vi "Test Exec.vi"(5 "Chunk Size":i32, 7 "Sample Rate":i32, 8 "Shape":T2, 9 "Frequency":T3, 10 "Offset":T3, 11 "Amplitude":T3) -> (3 "Out":T1)   [LabVIEW 2022 SP3]
uses:
  <extravilib>/ChannelInstances/Flex-dbl/))Channel.ctl
  <extravilib>/ChannelInstances/Flex-t'FGen.lvlib-Shape.ctl'/))Channel.ctl
  Users/Localization Tester/Documents/LabVIEW Data/IlluminatedG/FlexBlocks/Workers/FGen/Shape.ctl
  <extravilib>/ChannelInstances/Flex-c(dbl,dbl,a[.](dbl))/))Channel.ctl
  Users/Localization Tester/Documents/LabVIEW Data/IlluminatedG/FlexBlocks/Workers/FGen/State.ctl
  FlexBlocks Support/Worker Action.ctl
  Users/Localization Tester/Documents/LabVIEW Data/IlluminatedG/FlexBlocks/Workers/FGen/Init.ctl
  Users/Localization Tester/Documents/LabVIEW Data/IlluminatedG/FlexBlocks/Workers/FGen/Tags.ctl
  f1ba7f41-6067-463b-82d1-95e17fac6f2e.vi
  Users/Localization Tester/Documents/LabVIEW Data/IlluminatedG/FlexBlocks/Workers/FGen/Work.vi
  <extravilib>/ChannelInstances/Messenger-t'FlexBlocks Support.lvlib-Execution Events.ctl'/Instantiate.vi
  FlexBlocks Support/FlexBlocks Support.lvlib
  Users/Localization Tester/Documents/LabVIEW Data/IlluminatedG/FlexBlocks/Workers/FGen/FGen.lvlib
  <extravilib>/ChannelInstances/Flex-dbl.lvlib
  <extravilib>/ChannelInstances/Flex-t'FGen.lvlib-Shape.ctl'.lvlib
  <extravilib>/ChannelInstances/Flex-c(dbl,dbl,a[.](dbl)).lvlib
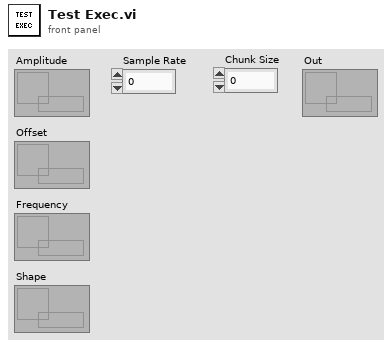
[diagram p1: front panel]
types:
  T1 = typedef "Flex-c(dbl,dbl,a[.](dbl)).lvlib/))Channel.ctl" = refnum<queue>
  T2 = typedef "Flex-t'FGen.lvlib-Shape.ctl'.lvlib/))Channel.ctl" = refnum<queue>
  T3 = typedef "Flex-dbl.lvlib/))Channel.ctl" = refnum<queue>
  T4 = typedef "FGen.lvlib/State.ctl" = cluster{"sampling info":cluster{"Fs":dbl, "#s":dbl}, "dx":dbl, "Delay":i32}
  T5 = typedef "Messenger-t'FlexBlocks Support.lvlib-Execution Events.ctl'.lvlib/))Channel.ctl" = refnum<queue>
  T6 = typedef "FlexBlocks Support.lvlib/Worker Block.ctl" = cluster{"Block Status":refnum<user-event>, "Command Queue":refnum<queue>, "Status":T7}
  T7 = typedef "FlexBlocks Support.lvlib/Block Status with Error.ctl" = cluster{"Block Status":T8, "Error":errorcluster}
  T8 = typedef "FlexBlocks Support.lvlib/Block Status.ctl" = cluster{"State":T9, "Next State":T9, "Runs":u32, "i":i32, "Init":bool, "Started":bool, "Closing":bool, "Step":bool, "Phase":T10, "Worker":string}
  T9 = typedef "FlexBlocks Support.lvlib/Block State.ctl" = enum16{"Idle", "Init", "Start", "Run", "Stop", "Close"}
  T10 = typedef "FlexBlocks Support.lvlib/Block Phase.ctl" = enum16{"N/A", "Read", "Work", "Write"}
  T11 = typedef "FlexBlocks Support.lvlib/Worker Action.ctl" = enum16{"Init", "Start", "Run", "Stop", "Close"}
  T12 = typedef "FGen.lvlib/Shape.ctl" = enum16{"Sine", "Square", "Triangle", "Saw"}
  T13 = typedef "FGen.lvlib/Init.ctl" = cluster{"Sample Rate":i32, "Chunk Size":i32}
  T14 = typedef "FGen.lvlib/Tags.ctl" = cluster{"Shape":T12, "Frequency":dbl, "Amplitude":dbl, "Offset":dbl}
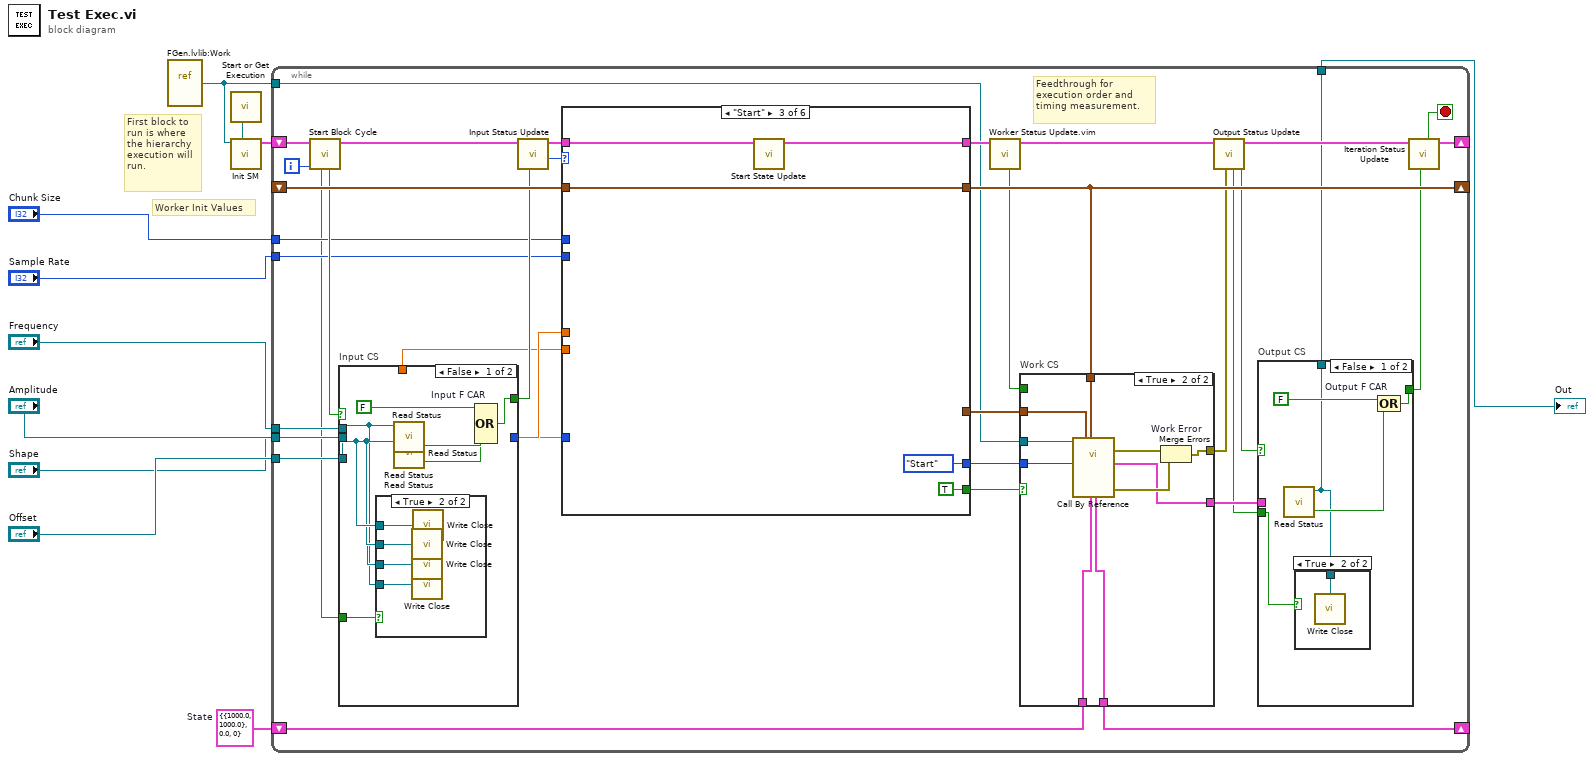
[diagram p0: block diagram]
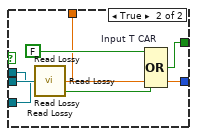
[diagram p3: hidden frame]
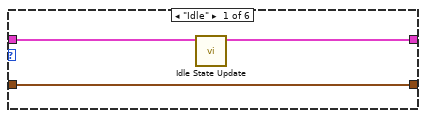
[diagram p4: hidden frame]
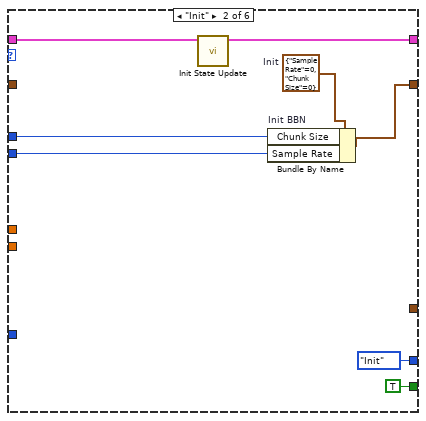
[diagram p5: hidden frame]
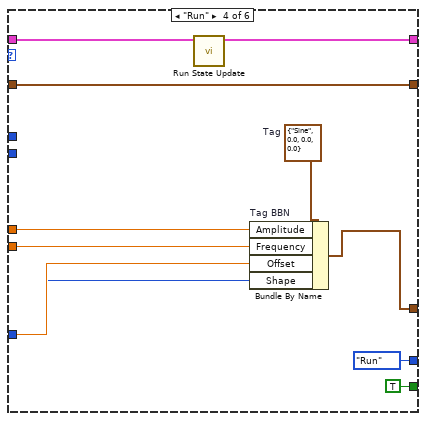
[diagram p6: hidden frame]
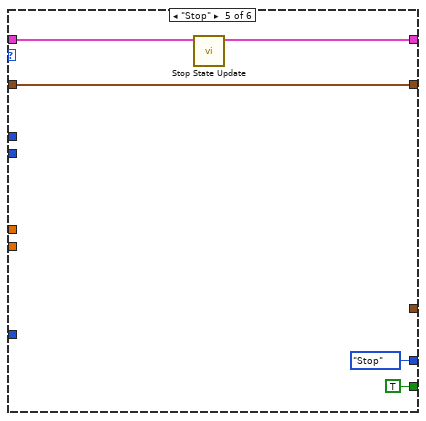
[diagram p7: hidden frame]
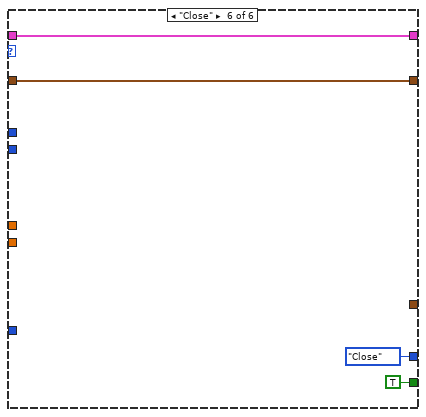
[diagram p8: hidden frame]
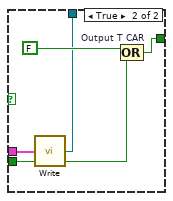
[diagram p10: hidden frame]
diagram:
  w11 = T4 {"sampling info"={"Fs"=1000.0, "#s"=1000.0}, "dx"=0.0, "Delay"=0}  # State
  # "First block to run is where the hierarchy execution will run."
  # "Worker Init Values"
  n1 = vi-ref "FGen.lvlib:Work.vi"() -> (w10:refnum<vi>)
  n2 = call "Start or Get Execution.vi"() -> ("Exec Events"=w9:T5)  [unwired: 11 in]
  n3 = call "Init SM.vi"("Exec Events"=w9, "Work VI"=w10) -> ("Worker Block"=w8:T6)  [unwired: 9 in]
  n4 = while {
    tunnel: w10 -> [w29]
    shift-right: [w48] -> _
    shift-left: w11 -> [w49]
    shift-right: [w34] -> _
    shift-left: w8 -> [w41]
    shift-right: [w45] -> _
    shift-left: _ -> [w46]
    tunnel: "Chunk Size" -> [w26]
    tunnel: "Sample Rate" -> [w25]
    tunnel: "Amplitude" -> [w24]
    tunnel: "Frequency" -> [w22]
    tunnel: "Offset" -> [w20]
    tunnel: "Shape" -> [w18]
    tunnel: [w16] -> w1
    i -> [w27]
    stop <- w32 stop-if-true
    # "Feedthrough for execution order and timing measurement."
    n5 = call "Start Block Cycle.vi"("i"=w27, "Worker Block In"=w41) -> ("Worker Block"=w40:T6, "Do Read"=w43:bool, "Close"=w14:bool)  [unwired: 7 in]
    n6 = case "Input CS" shown="False" w43 {
      tunnel: [w60 w78] -> w39
      tunnel: w24 -> [w50 w76]
      tunnel: [_ w74] -> w23
      tunnel: w22 -> [w51 w73]
      tunnel: [_ w71] -> w21
      tunnel: w20 -> [w52 w70]
      tunnel: [_ w68] -> w19
      tunnel: w18 -> [w53 w67]
      tunnel: [_ w65] -> w17
      tunnel: w14 -> [w54 _]
      frame False {
        n7 = case shown="True" w54 {
          tunnel: w53 -> [_ w64]
          tunnel: w52 -> [_ w63]
          tunnel: w51 -> [_ w62]
          tunnel: w50 -> [_ w61]
          frame False {
          }
          frame True {
            n8 = call <extravilib>:"Write Close.vi"("FlexChannel"=w63) -> ()
            n9 = call <extravilib>:"Write Close.vi"("FlexChannel"=w62) -> ()
            n10 = call <extravilib>:"Write Close.vi"("FlexChannel"=w61) -> ()
            n11 = call <extravilib>:"Write Close.vi"("FlexChannel"=w64) -> ()
          }
        }
        n12 = call <extravilib>:"Read Status.vi"("channel"=w50) -> ("Closed?"=w58:bool)  [unwired: 4 in, 6 out]
        n13 = call <extravilib>:"Read Status.vi"("channel"=w53) -> ("Closed?"=w55:bool)  [unwired: 4 in, 6 out]
        n14 = call <extravilib>:"Read Status.vi"("channel"=w52) -> ("Closed?"=w56:bool)  [unwired: 4 in, 6 out]
        n15 = call <extravilib>:"Read Status.vi"("channel"=w51) -> ("Closed?"=w57:bool)  [unwired: 4 in, 6 out]
        n16 = Compound Arithmetic op=OR "Input F CAR"(FALSE, w58, w57, w56, w55) -> (w60:bool)
      }
      frame True {
        n17 = call <extravilib>:"Read Lossy.vi"("FlexChannel"=w67) -> ("Value"=w65:T12, "Closed?"=w66:bool)  [unwired: 4 in, 3 out]
        n18 = call <extravilib>:"Read Lossy.vi"("FlexChannel"=w70) -> ("Value"=w68:dbl, "Closed?"=w69:bool)  [unwired: 4 in, 3 out]
        n19 = call <extravilib>:"Read Lossy.vi"("FlexChannel"=w73) -> ("Value"=w71:dbl, "Closed?"=w72:bool)  [unwired: 4 in, 3 out]
        n20 = call <extravilib>:"Read Lossy.vi"("FlexChannel"=w76) -> ("Value"=w74:dbl, "Closed?"=w75:bool)  [unwired: 4 in, 3 out]
        n21 = Compound Arithmetic op=OR "Input T CAR"(FALSE, w75, w72, w69, w66) -> (w78:bool)
      }
    }
    n22 = call "Input Status Update.vi"("Input Closed?"=w39, "Worker Block In"=w40) -> ("Block State"=w42:T9, "Worker Block"=w38:T6)  [unwired: 8 in]
    n23 = case shown="\"Start\"" w42 {
      tunnel: [_ _ _ w103 _ _] -> w47
      tunnel: [w81 w88 w94 w105 w110 w114] -> w45
      tunnel: w46 -> [w81 _ w94 w105 w110 w114]
      tunnel: [w79 w86 w92 w99 w106 w111] -> w37
      tunnel: w38 -> [w80 w87 w93 w100 w107 w111]
      tunnel: [_ Worker_Action."Init" ("Action") Worker_Action."Start" ("Action") Worker_Action."Run" ("Action") Worker_Action."Stop" ("Action") Worker_Action."Close" ("Action")] -> w31
      tunnel: [_ TRUE TRUE TRUE TRUE TRUE] -> w30
      tunnel: w26 -> [_ w83 _ _ _ _]
      tunnel: w25 -> [_ w82 _ _ _ _]
      tunnel: w23 -> [_ _ _ w98 _ _]
      tunnel: w21 -> [_ _ _ w97 _ _]
      tunnel: w19 -> [_ _ _ w96 _ _]
      tunnel: w17 -> [_ _ _ w95 _ _]
      frame "Idle" {
        n24 = call "Idle State Update.vi"("Worker Block In"=w80) -> ("Worker Block"=w79:T6)  [unwired: 10 in]
      }
      frame "Init" {
        w89 = T13 {"Sample Rate"=0, "Chunk Size"=0}  # Init
        n25 = call "Init State Update.vi"("Worker Block In"=w87) -> ("Worker Block"=w86:T6)  [unwired: 10 in]
        n26 = Bundle By Name "Init BBN"(cluster=w89, "Chunk Size"=w83, "Sample Rate"=w82) -> (w88:T13)
      }
      frame "Start" {
        n27 = call "Start State Update.vi"("Worker Block In"=w93) -> ("Worker Block"=w92:T6)  [unwired: 10 in]
      }
      frame "Run" {
        w104 = T14 {"Shape"=enum."Sine", "Frequency"=0.0, "Amplitude"=0.0, "Offset"=0.0}  # Tag
        n28 = call "Run State Update.vi"("Worker Block In"=w100) -> ("Worker Block"=w99:T6)  [unwired: 10 in]
        n29 = Bundle By Name "Tag BBN"(cluster=w104, "Amplitude"=w98, "Frequency"=w97, "Offset"=w96, "Shape"=w95) -> (w103:T14)
      }
      frame "Stop" {
        n30 = call "Stop State Update.vi"("Worker Block In"=w107) -> ("Worker Block"=w106:T6)  [unwired: 10 in]
      }
      frame "Close" {
      }
    }
    n31 = call "Worker Status Update.vim"("Worker Block In"=w37) -> ("Worker Block"=w36:T6, "Flow Control"=w28:bool)  [unwired: 9 in]
    n32 = case "Work CS" shown="True" w30 {
      tunnel: w29 -> [_ w137]
      tunnel: w49 -> [w127 w134]
      tunnel: [w127 w133] -> w48
      tunnel: w47 -> [_ w131]
      tunnel: w31 -> [_ w130]
      tunnel: w45 -> [_ w132]
      tunnel: [_ w135] -> w44
      tunnel: w28 -> [_ _]
      tunnel: [_ w128] -> w15
      frame False {
      }
      frame True {
        n33 = call-by-ref "?"(reference=w137, "Action"=w130, "Tags"=w131, "Init"=w132, "State in"=w134) -> (error out=w136:errorcluster, "State out"=w133:T4, "Out"=w128:cluster{dbl, "dx":dbl, "Y":dbl[]}, "Error"=w129:errorcluster)  [unwired: 14 in, 1 out]
        n34 = Merge Errors "Work Error"(w136, w129) -> (w135:errorcluster)
      }
    }
    n35 = call "Output Status Update.vi"("Worker Error"=w44, "Worker Block In"=w36) -> ("Write Outputs"=w13:bool, "Worker Block"=w35:T6, "Close?"=w12:bool)  [unwired: 7 in]
    n36 = case "Output CS" shown="False" w13 {
      tunnel: [w119 w126] -> w33
      tunnel: [w116 w124] -> w16
      tunnel: w15 -> [_ w122]
      tunnel: w12 -> [w115 w121]
      frame False {
        n37 = call <extravilib>:"Read Status.vi"() -> ("Closed?"=w117:bool, "channel"=w116:T1)  [unwired: 4 in, 6 out]
        n38 = case shown="True" w115 {
          tunnel: w116 -> [_ w120]
          frame False {
          }
          frame True {
            n39 = call <extravilib>:"Write Close.vi"("FlexChannel"=w120) -> ()
          }
        }
        n40 = Compound Arithmetic op=OR "Output F CAR"(FALSE, w117) -> (w119:bool)
      }
      frame True {
        n41 = call <extravilib>:"Write.vi"("element"=w122, "Close? (F)"=w121) -> ("channel"=w124:T1, "Closed?"=w123:bool)  [unwired: 5 in, 1 out]
        n42 = Compound Arithmetic op=OR "Output T CAR"(FALSE, w123) -> (w126:bool)
      }
    }
    n43 = call "Iteration Status Update.vi"("Output Closed?"=w33, "Worker Block In"=w35) -> ("Worker Block"=w34:T6, "Stop Block"=w32:bool)  [unwired: 8 in]
  }
  "Out" <- w1
